vi "start_stimulation.vi"(8 "error in (no error)":errorcluster, 11 "DL090503StimulatorScaffold in":refnum<class "StimulatorAK101022TCP.lvclass">) -> (0 "error out":errorcluster, 3 "DL090503StimulatorScaffold out":refnum<class "StimulatorAK101022TCP.lvclass">)   [LabVIEW 2010, in "StimulatorAK101022TCP.lvclass"]
uses:
  StimulatorAK101022TCP.lvclass
  StimulatorDL090503Scaffold/StimulatorDL090503Scaffold/StimulatorDL090503Scaffold.lvclass
  StimulatorAK101022TCP.lvclass/StimulatorAK101022TCP.ctl
  StringGenerator/GenericStringGenerator/GenericStringGenerator/GenericStringGenerator.lvclass
  common/classes/NoteBook/Notebook/Notebook.lvclass
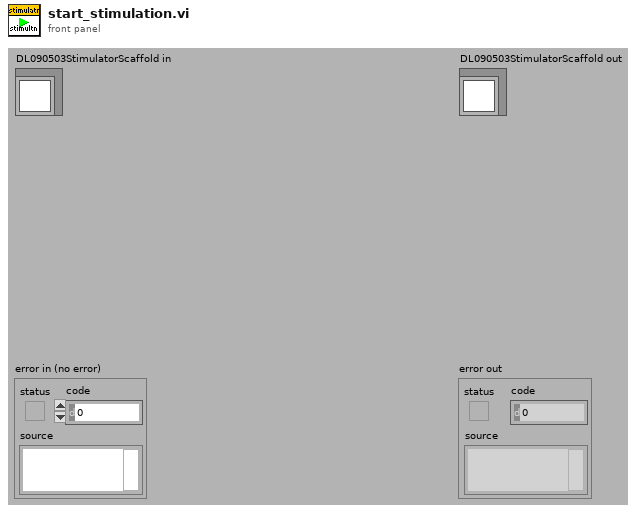
[diagram p1: front panel]
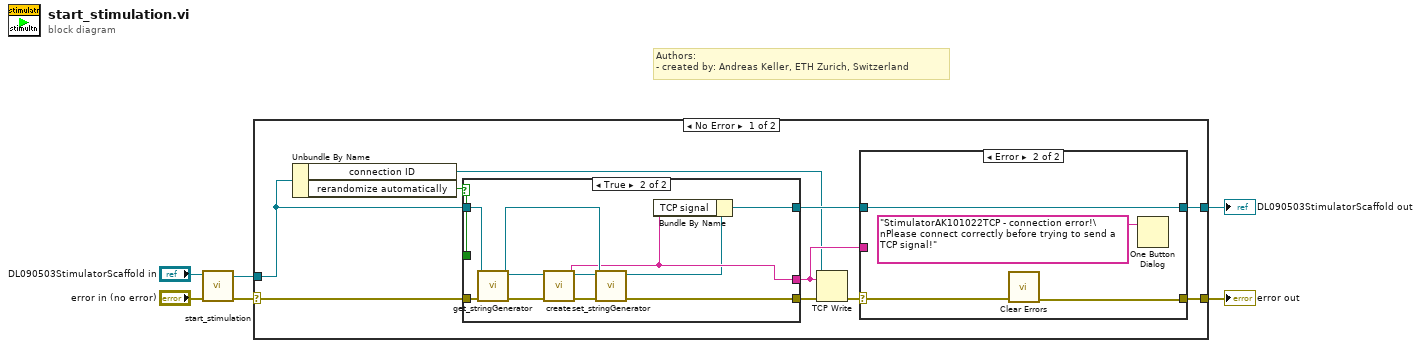
[diagram p0: block diagram]
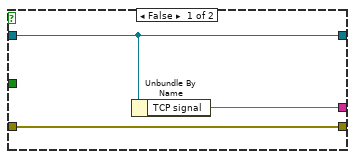
[diagram p2: hidden frame]
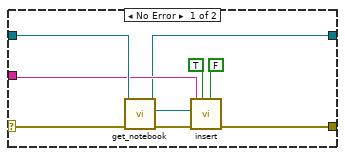
[diagram p3: hidden frame]
diagram:
  # "Authors: \n- created by: Andreas Keller, ETH Zurich, Switzerland"
  n1 = call-parent "start_stimulation.vi"("error in (no error)"="error in (no error)", "DL090503StimulatorScaffold in"="DL090503StimulatorScaffold in") -> ("error out"=w4:errorcluster, "DL090503StimulatorScaffold out"=w1:refnum<class "StimulatorAK101022TCP.lvclass">)  [unwired: 8 in]
  n2 = case shown="No Error" w4 {
    selector: w4 -> [w13 w45]
    tunnel: [w15 w45] -> w3
    tunnel: [w14 w44] -> w2
    tunnel: w1 -> [w11 w44]
    frame No Error {
      n3 = Unbundle By Name(w11) -> ("connection ID"=w7:refnum<k5>, "rerandomize automatically"=w8:bool)
      n4 = case shown="True" w8 {
        tunnel: w13 -> [w19 w30]
        tunnel: [w19 w24] -> w12
        tunnel: w11 -> [w18 w29]
        tunnel: [w18 w22] -> w10
        tunnel: [w17 w21] -> w9
        tunnel: w8 -> [_ _]
        frame False {
          n5 = Unbundle By Name(w18) -> ("TCP signal"=w17:string)
        }
        frame True {
          n6 = call-dynamic "get_stringGenerator.vi"("error in (no error)"=w30, "StimulatorAK101022TCP in"=w29) -> ("error out"=w28:errorcluster, "stringGenerator"=w27:refnum<class "GenericStringGenerator.lvclass">, "StimulatorAK101022TCP out"=w23:refnum<class "StimulatorAK101022TCP.lvclass">)  [unwired: 7 in]
          n7 = call-dynamic "create.vi"("error in (no error)"=w28, "GenericStringGenerator in"=w27) -> ("error out"=w25:errorcluster, "String"=w21:string, "GenericStringGenerator out"=w26:refnum<class "GenericStringGenerator.lvclass">)  [unwired: 7 in]
          n8 = call-dynamic "set_stringGenerator.vi"("error in (no error)"=w25, "subcomponents.stringGenerator"=w26, "StimulatorAK101022TCP in"=w23) -> ("error out"=w24:errorcluster, "StimulatorAK101022TCP out"=w20:refnum<class "StimulatorAK101022TCP.lvclass">)  [unwired: 7 in]
          n9 = Bundle By Name(cluster=w20, "TCP signal"=w21) -> (w22:refnum<class "StimulatorAK101022TCP.lvclass">)
        }
      }
      n10 = TCP Write(connection ID=w7, data in=w9, error in (no error)=w12) -> (error out=w16:errorcluster)  [unwired: 1 in, 2 out]
      n11 = case shown="Error" w16 {
        selector: w16 -> [w38 w43]
        tunnel: [w32 w42] -> w15
        tunnel: w10 -> [w36 w40]
        tunnel: [w31 w40] -> w14
        tunnel: w9 -> [w35 _]
        frame No Error {
          n12 = call-dynamic "get_notebook.vi"("error in (no error)"=w38, "GenericComponent in"=w36) -> ("error out"=w39:errorcluster, "notebook"=w37:refnum<class "Notebook.lvclass">, "GenericComponent out"=w31:refnum<class "StimulatorAK101022TCP.lvclass">)  [unwired: 7 in]
          n13 = call "insert.vi"("add line break after?"=FALSE, "add line break before?"=TRUE, "error in (no error)"=w39, "string"=w35, "Notebook in"=w37) -> ("error out"=w32:errorcluster)  [unwired: 5 in, 1 out]
        }
        frame Error {
          n14 = call <vilib>:"Clear Errors.vi"("error in (no error)"=w43) -> ("error out"=w42:errorcluster)  [unwired: 6 in]
          n15 = One Button Dialog(message="StimulatorAK101022TCP - connection error!\nPlease connect correctly before trying to send a TCP signal!") -> ()  [unwired: 1 in, 1 out]
        }
      }
    }
    frame Error {
    }
  }
  "error out" <- w3
  "DL090503StimulatorScaffold out" <- w2
